vi "Calibrate Force.vi"(8 "error in (no error)":errorcluster, 9 "DAQ  Channels In":T1={"Force Transducer: Left"="Dev1/ai6", "Force Transducer: Right "="Dev1/ai8", "EMG: Left"="", "EMG: Right"="", "Potentiometer: Left"="", "Potentiometer: Right"=""}, 10 "rate":dbl=1000.0 format="%0.2f", 11 "NI Force Task in":refnum<class "NI Force Task.lvclass">) -> (0 "error out":errorcluster, 3 "NI Force Task out":refnum<class "NI Force Task.lvclass">)   [LabVIEW 2020, in "NI Force Task.lvlib" / "NI Force Task.lvclass"]
uses:
  NI Force Task.lvclass
  NI Force Task.lvclass/NI Force Task.ctl
  <vilib>/DAQmx/create/channels.llb/DAQmx Create Channel (AI-Voltage-Basic).vi
  <vilib>/DAQmx/configure/timing.llb/DAQmx Timing (Sample Clock).vi
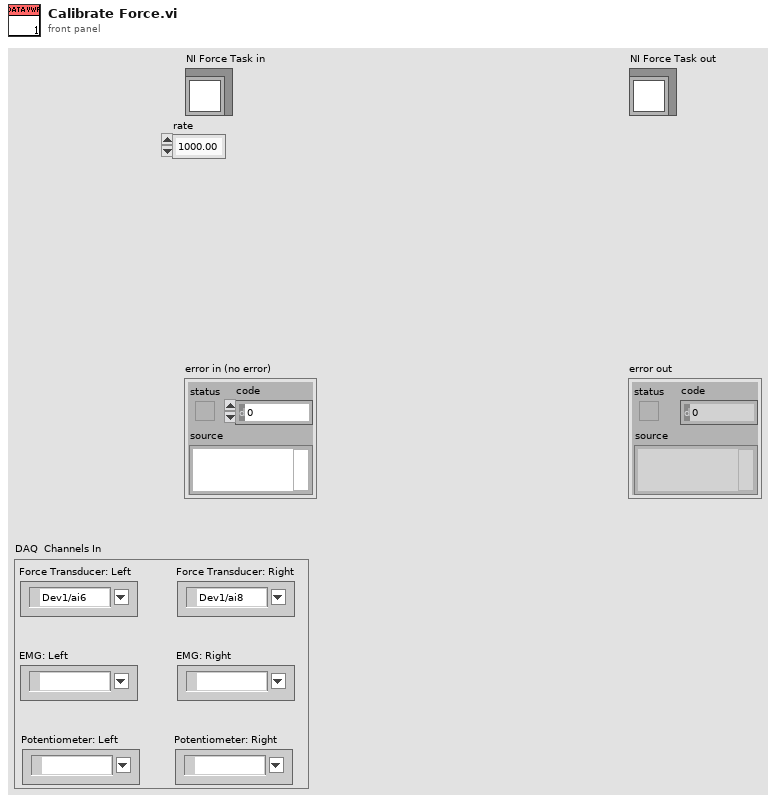
[diagram p1: front panel]
types:
  T1 = cluster{"Force Transducer: Left":tag, "Force Transducer: Right ":tag, "EMG: Left":tag, "EMG: Right":tag, "Potentiometer: Left":tag, "Potentiometer: Right":tag}
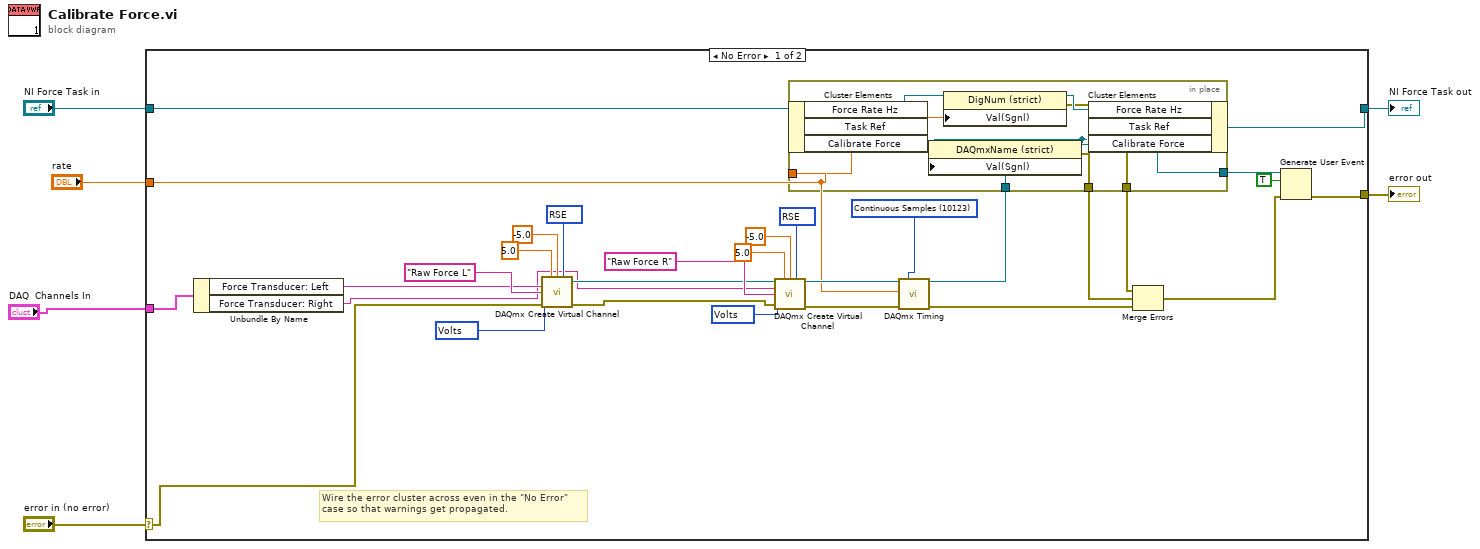
[diagram p0: block diagram]
diagram:
  n1 = case shown="No Error" "error in (no error)" {
    selector: "error in (no error)" -> [w7 w47]
    tunnel: [w8 w47] -> w5
    tunnel: [w17 w46] -> w3
    tunnel: "NI Force Task in" -> [w18 w46]
    tunnel: "DAQ  Channels In" -> [w22 _]
    tunnel: "rate" -> [w16 _]
    frame No Error {
      w21 = 10123 items=["Finite Samples"=10178, "Continuous Samples"=10123, "Hardware Timed Single Point"=12522] ("sample mode")
      w27 = 10348 items=["Volts"=10348, "From Custom Scale"=10065] ("units")
      w31 = 10083 items=["Default"=-1, "RSE"=10083, "NRSE"=10078, "Differential"=10106, "Pseudodifferential"=12529] ("input terminal configuration")
      w32 = 10348 items=["Volts"=10348, "From Custom Scale"=10065] ("units")
      w36 = 10083 items=["Default"=-1, "RSE"=10083, "NRSE"=10078, "Differential"=10106, "Pseudodifferential"=12529] ("input terminal configuration")
      # "Wire the error cluster across even in the \"No Error\"\ncase so that warnings get propagated."
      n2 = Unbundle By Name(w22) -> ("Force Transducer: Left"=w24:tag, "Force Transducer: Right"=w23:tag)
      n3 = call-poly <vilib>:"DAQmx Create Virtual Channel.vi"("maximum value"=5.0, "minimum value"=-5.0, "input terminal configuration"=w36, "physical channels"=w24, "name to assign"="Raw Force L", "units"=w32, "error in"=w7) -> ("task out"=w26:refnum<k21>, "error out"=w25:errorcluster)  [unwired: 7 in]
      n4 = call-poly <vilib>:"DAQmx Create Virtual Channel.vi"("task in"=w26, "maximum value"=5.0, "minimum value"=-5.0, "input terminal configuration"=w31, "physical channels"=w23, "name to assign"="Raw Force R", "units"=w27, "error in"=w25) -> ("task out"=w20:refnum<k21>, "error out"=w19:errorcluster)  [unwired: 6 in]
      n5 = call-poly <vilib>:"DAQmx Timing.vi"("task/channels in"=w20, "sample mode"=w21, "rate"=w16, "error in"=w19) -> ("task out"=w15:refnum<k21>, "error out"=w12:errorcluster)  [unwired: 10 in]
      n6 = in-place {
        in-place-border: w16 -> [w41]
        in-place-border: w15 -> [w40]
        in-place-border: [w39] -> w14
        in-place-border: [w38] -> w13
        in-place-border: [w37] -> w11
        n7 = in-place-cluster #1(w18) -> ("Force Rate Hz"=w45:refnum<vi>, "Task Ref"=w43:refnum<vi>, "Calibrate Force"=w37:refnum<user-event>)
        n8 = property class="DAQmxName (strict)"(reference=w43, "Val(Sgnl)"=w40) -> (reference out=w42:refnum<vi>, error out=w38:errorcluster)  [unwired: 1 in]
        n9 = property class="DigNum (strict)"(reference=w45, "Val(Sgnl)"=w41) -> (reference out=w44:refnum<vi>, error out=w39:errorcluster)  [unwired: 1 in]
        n10 = in-place-cluster #1("Force Rate Hz"=w44, "Task Ref"=w42, "Calibrate Force"=w37) -> (w17:refnum<class "NI Force Task.lvclass">)
      }
      n11 = Merge Errors(w14, w13, w12) -> (w9:errorcluster)
      n12 = Generate User Event(user event=w11, event data cluster=TRUE ("event data"), error in=w9) -> (error out=w8:errorcluster)  [unwired: 1 in, 1 out]
    }
    frame Error {
    }
  }
  "error out" <- w5
  "NI Force Task out" <- w3
